vi "Within limits.vi"(10 "Limits":cluster{"Min":i64, "Max":i64}, 11 "Rational Number in":refnum<class "Rational Number.lvclass">) -> (3 "In Limits?":bool)   [LabVIEW 2021, in "Rational Number.lvclass"]
uses:
  Rational Number.lvclass
  Rational Number.lvclass/Rational Number.ctl
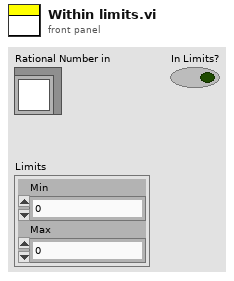
[diagram p1: front panel]
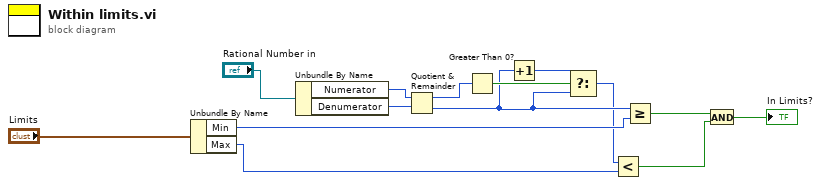
[diagram p0: block diagram]
diagram:
  n1 = Unbundle By Name("Limits") -> ("Min"=w10:i64, "Max"=w9:i64)
  n2 = Unbundle By Name("Rational Number in") -> ("Numerator"=w12:i64, "Denumerator"=w11:i64)
  n3 = Quotient & Remainder(x=w12, y=w11) -> (x-y*floor(x/y)=w5:i64, floor(x/y)=w2:i64)
  n4 = Greater Than 0?(x=w5) -> (x > 0?=w4:bool)
  n5 = Increment(x=w2) -> (x+1=w3:i64)
  n6 = Select(t=w3, s=w4, f=w2) -> (s? t:f=w1:i64)
  n7 = Less?(x=w1, y=w9) -> (x < y?=w8:bool)
  n8 = Greater Or Equal?(x=w2, y=w10) -> (x >= y?=w6:bool)
  n9 = And(x=w6, y=w8) -> (x .and. y?=→"In Limits?":bool)
